vi "addcase.vi"() -> ()   [LabVIEW 2021]
uses:
  addcaase1.ctl
  addcase2.ctl
panel:
  out "train coming to point (500m before the cross)":i32
  out "speed of train":string
  out "Traffic":string
  out "Traffic condition":string
  out "train":string
  out "Number of Car 2":dbl
  out "Stop of traffic":i32
  out "Wait Time for Train":i32
  out "Number of Car":dbl
  in  "stop":bool
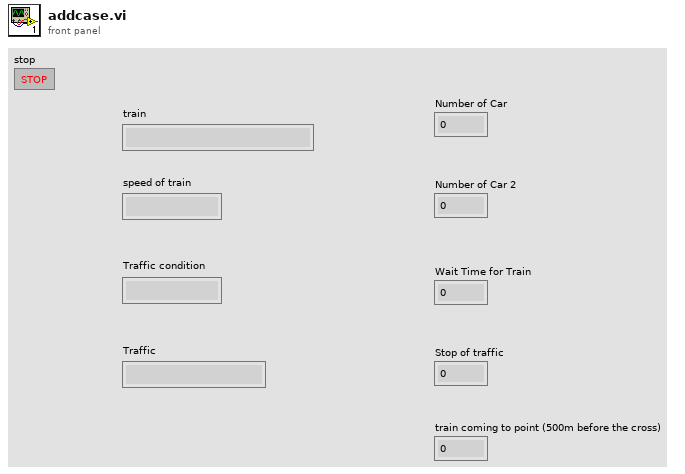
[diagram p1: front panel]
types:
  T1 = typedef "addcase2.ctl" = enum16{"Heavytraincrossing", "Heavytrafficwait", "Heavytraindepature", "Heavytrainwait", "Normal"}
  T2 = typedef "addcaase1.ctl" = enum16{"down", "traffice wait", "train departure", "up"}
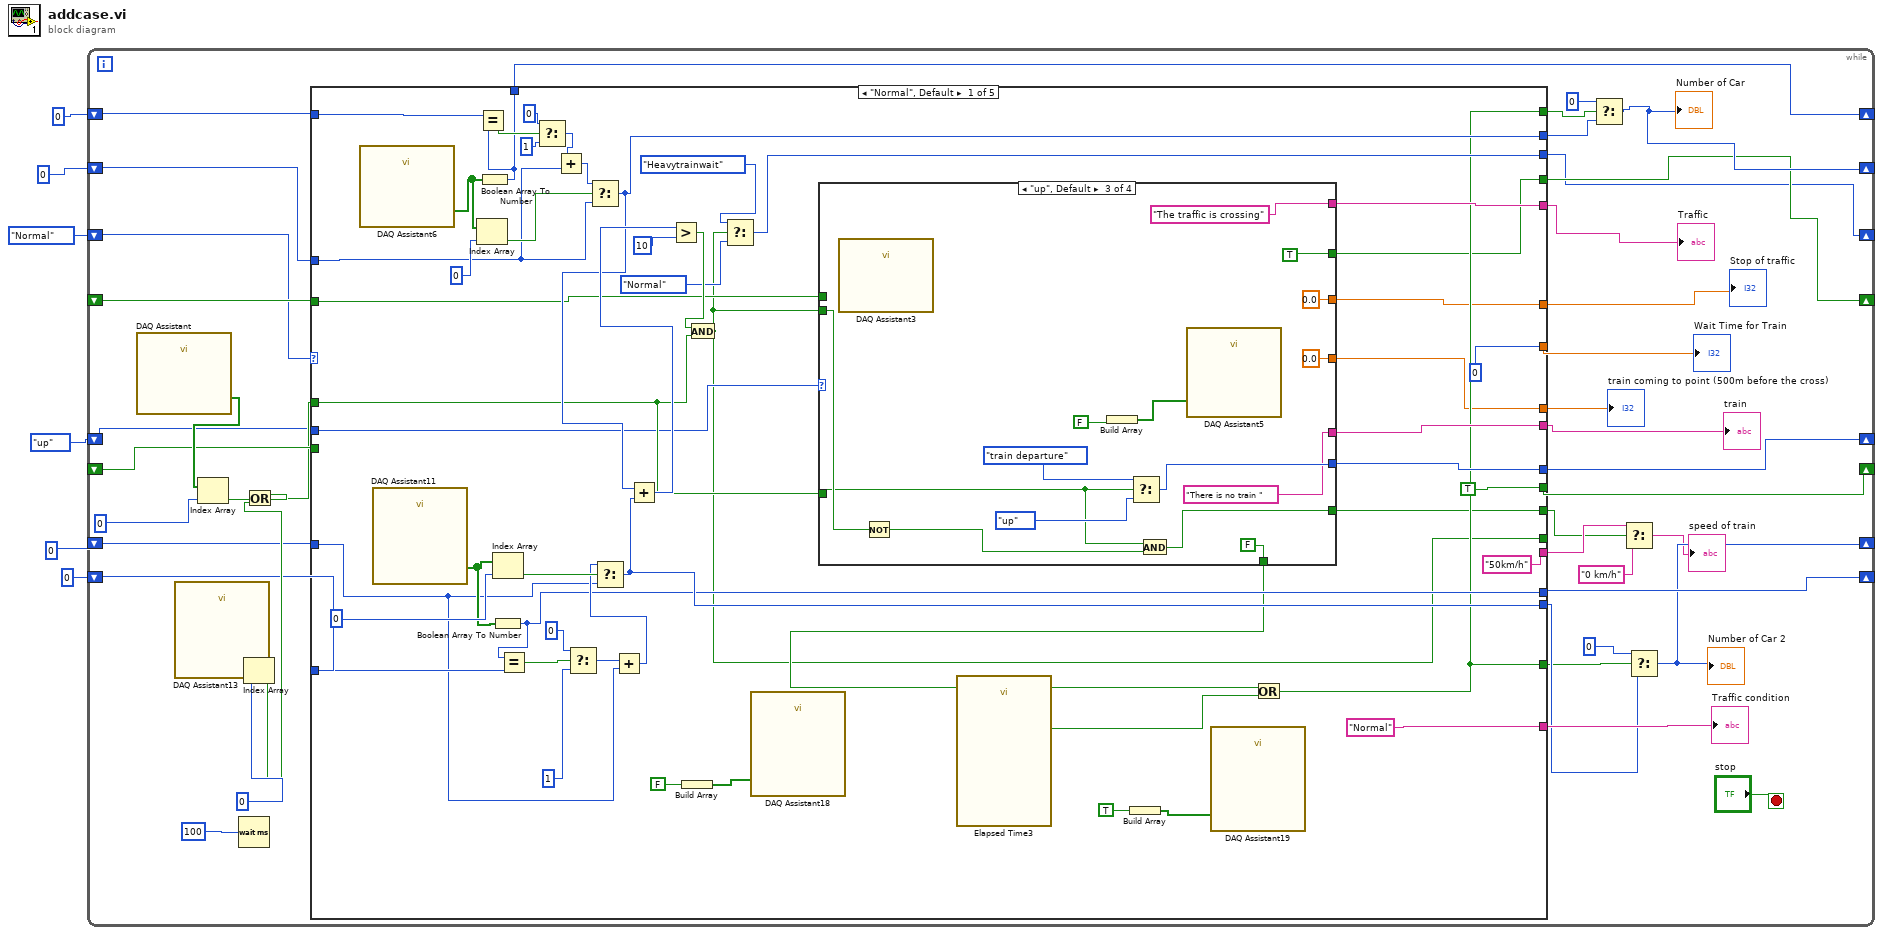
[diagram p0: block diagram]
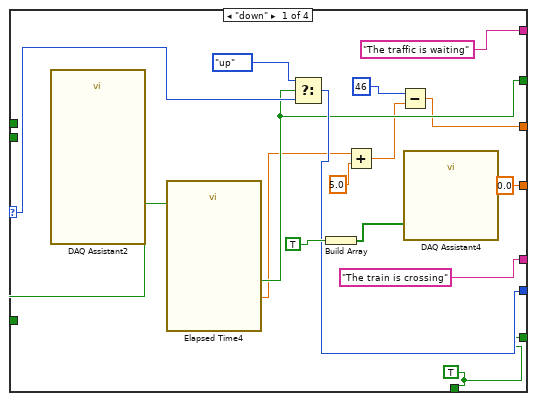
[diagram p2: hidden frame]
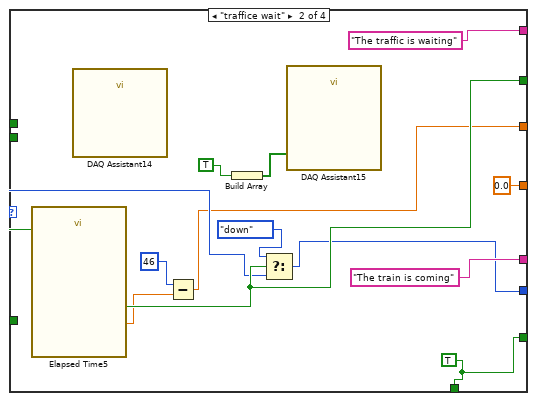
[diagram p3: hidden frame]
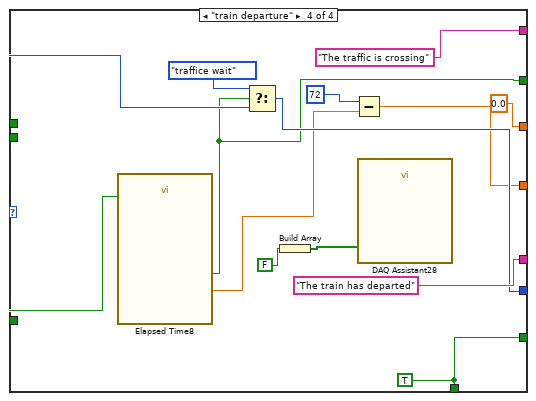
[diagram p4: hidden frame]
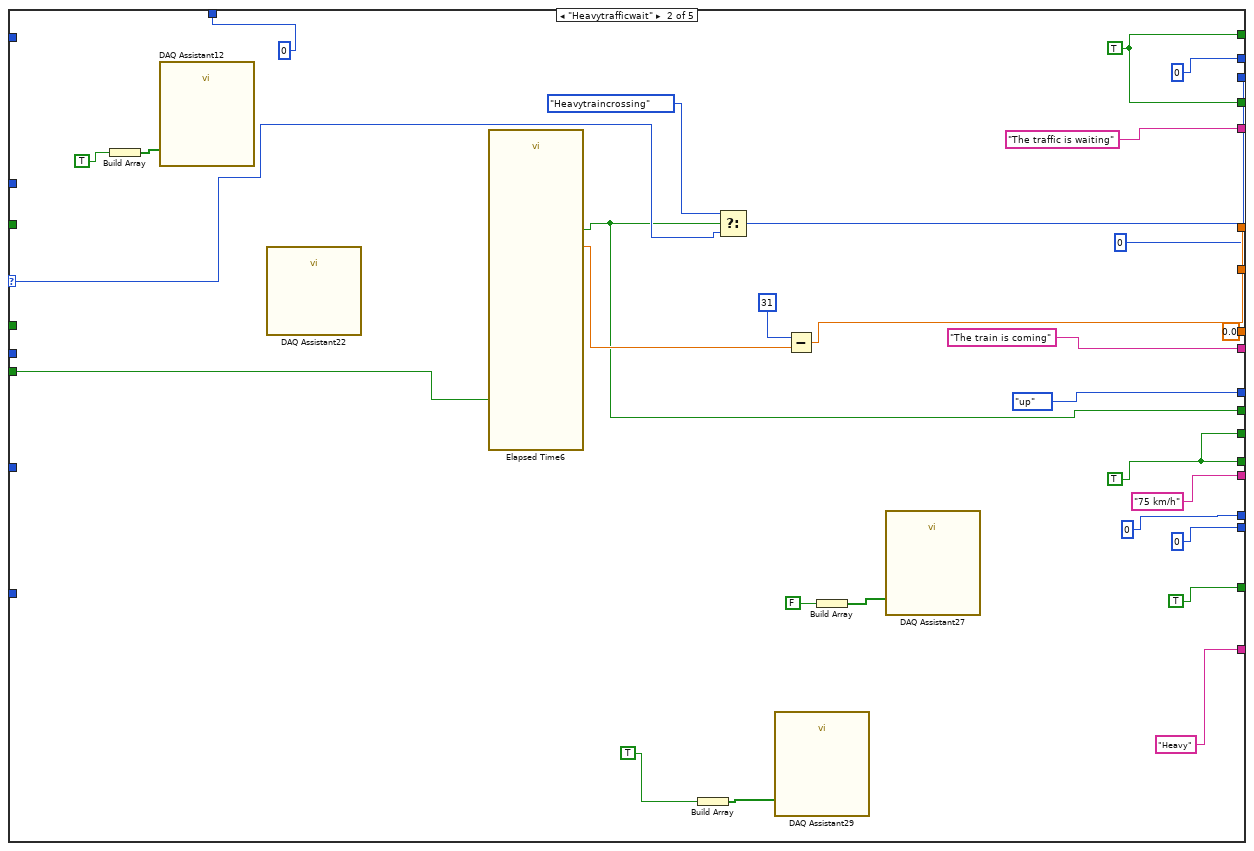
[diagram p5: hidden frame]
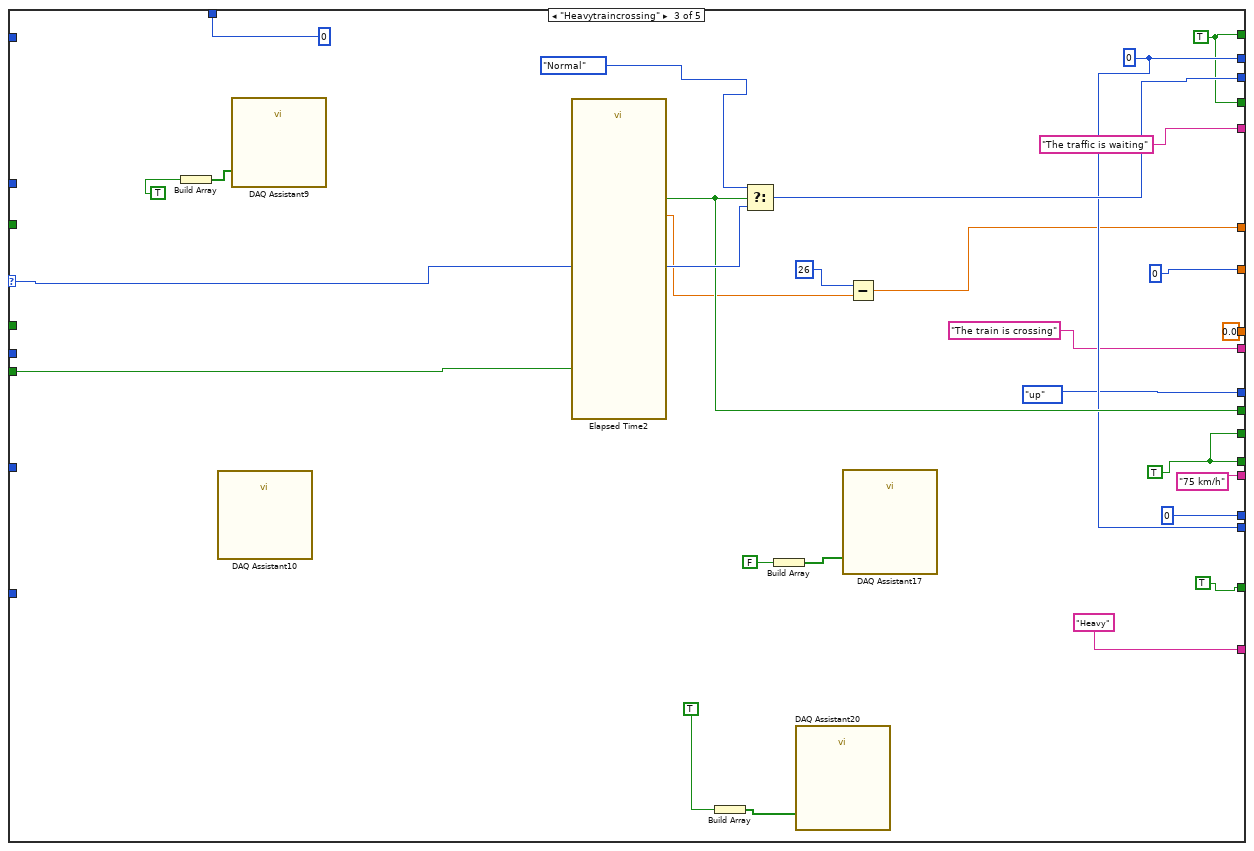
[diagram p6: hidden frame]
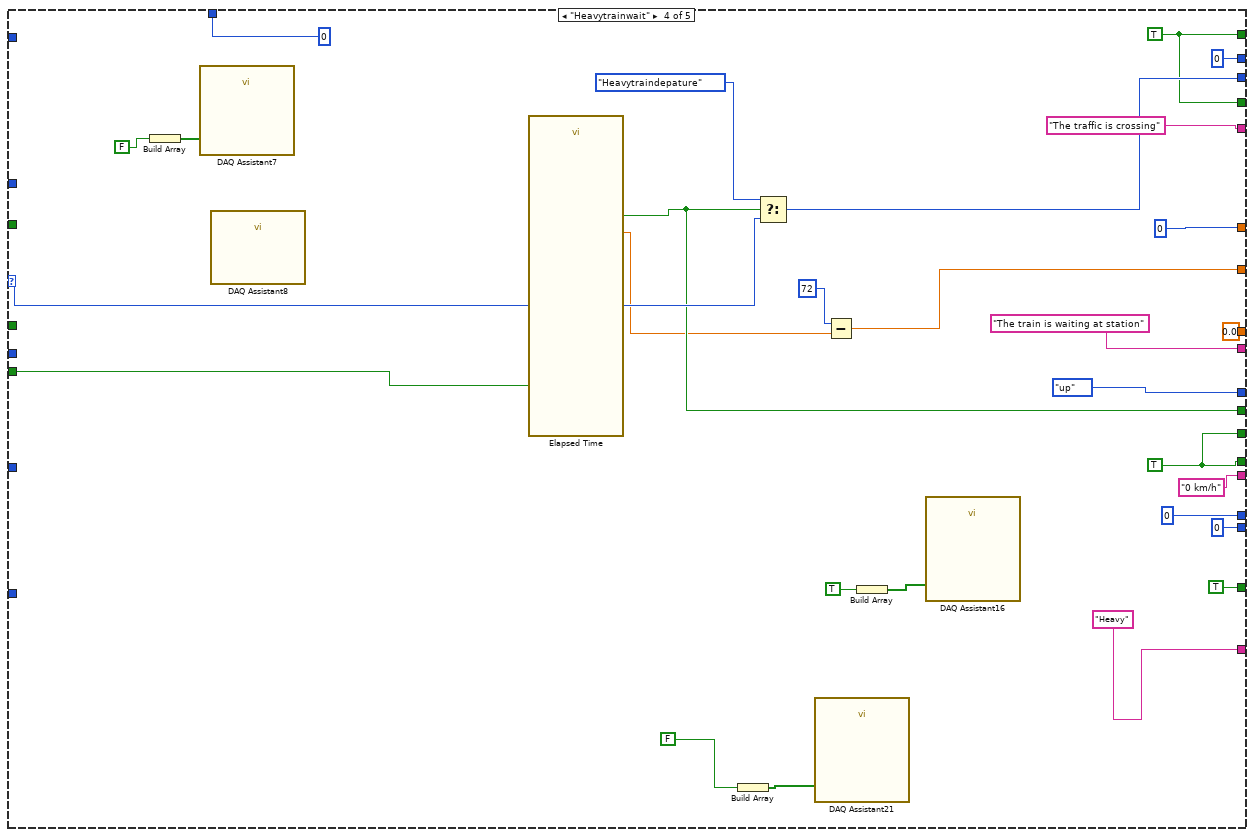
[diagram p7: hidden frame]
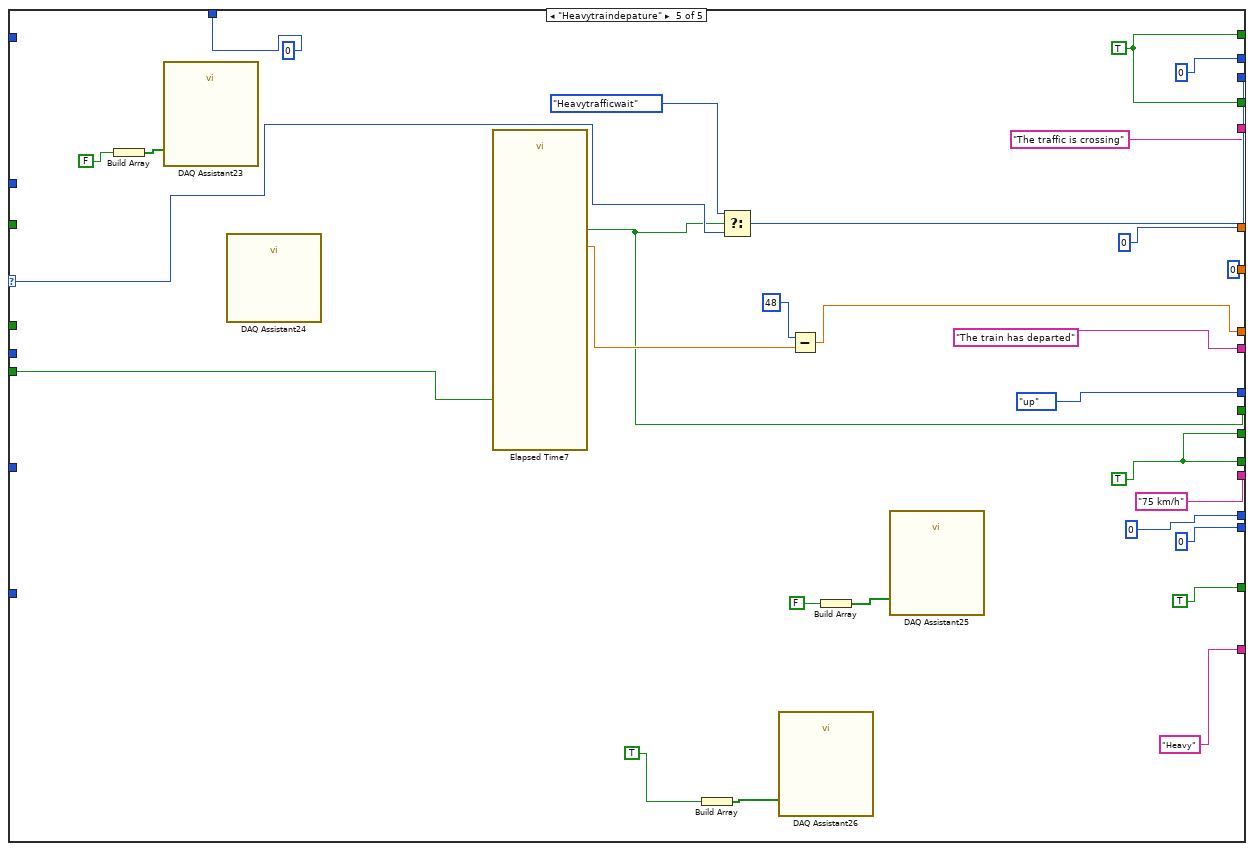
[diagram p8: hidden frame]
diagram:
  n1 = while {
    shift-right: [w22] -> _
    shift-left: 0 -> [w35]
    shift-right: [w42] -> _
    shift-left: _ -> [w41]
    shift-right: [w26] -> _
    shift-left: 0 -> [w34]
    shift-right: [w24] -> _
    shift-left: 0 ("index") -> [w33]
    shift-right: [w31] -> _
    shift-left: 0 ("index") -> [w32]
    shift-right: [w20] -> _
    shift-left: _ -> [w19]
    shift-right: [w14] -> _
    shift-left: addcaase1."up" -> [w15]
    shift-right: [w11] -> _
    shift-left: addcase2."Normal" -> [w12]
    stop <- "stop" stop-if-true
    n2 = call "DAQ Assistant"() -> ("data"=w46:bool[])  [unwired: 17 in, 2 out]
    n3 = call "DAQ Assistant13"() -> ("data"=w39:bool[])  [unwired: 17 in, 2 out]
    n4 = Index Array(array=w46, index=0) -> (element=w38:bool)
    n5 = Wait (ms)(milliseconds to wait=100) -> ()  [unwired: 1 out]
    n6 = Index Array(array=w39, index=0) -> (element=w37:bool)
    n7 = Or(x=w38, y=w37) -> (x .or. y?=w29:bool)
    n8 = case shown="\"Normal\", Default" w12 {
      selector: w12 -> [_ w175 w211 w239 w256]
      tunnel: w29 -> [w65 _ _ _ _]
      tunnel: [w98 w160 w210 w240 w255] -> w11
      tunnel: w35 -> [w78 _ _ _ _]
      tunnel: [w92 0 w206 0 0] -> w23
      tunnel: [w61 w167 w193 0 0] -> w44
      tunnel: [0 0 0 w221 0] -> w43
      tunnel: [TRUE w174 w208 w237 w254] -> w42
      tunnel: w41 -> [_ w177 w207 w236 w249]
      tunnel: w34 -> [w70 _ _ _ _]
      tunnel: [w93 0 w206 0 0] -> w27
      tunnel: w33 -> [w90 _ _ _ _]
      tunnel: [w85 u32 0 ("index") u32 0 ("index") u32 0 ("index") u32 0 ("index")] -> w24
      tunnel: [w84 addcaase1."up" addcaase1."up" addcaase1."up" addcaase1."up"] -> w14
      tunnel: w32 -> [w71 _ _ _ _]
      tunnel: [w72 u32 0 u32 0 u32 0 u32 0] -> w31
      tunnel: ["Normal" "Heavy" "Heavy" "Heavy" "Heavy"] -> w30
      tunnel: [w68 "The train is coming" "The train is crossing" "The train is waiting at station" "The train has departed"] -> w17
      tunnel: [w67 "The traffic is waiting" "The traffic is waiting" "The traffic is crossing" "The traffic is crossing"] -> w18
      tunnel: [w48 w159 w187 w214 w242] -> _
      tunnel: [w62 TRUE TRUE TRUE TRUE] -> w16
      tunnel: [w62 w163 w197 w225 w247] -> w21
      tunnel: [w60 w163 w197 w225 w247] -> w20
      tunnel: w19 -> [w59 _ _ _ _]
      tunnel: ["50km/h" "75 km/h" "75 km/h" "0 km/h" "75 km/h"] -> w10
      tunnel: w15 -> [w53 _ _ _ _]
      tunnel: [w52 0.0 ("Elapsed Time (s)") 0.0 ("Elapsed Time (s)") 0.0 ("Elapsed Time (s)") w244] -> w13
      tunnel: [w49 w159 w187 w214 w242] -> w8
      frame "Normal", Default {
        n9 = call "DAQ Assistant6"() -> ("data"=w88:bool[])  [unwired: 17 in, 2 out]
        n10 = call "DAQ Assistant11"() -> ("data"=w83:bool[])  [unwired: 17 in, 2 out]
        n11 = Index Array(array=w88, index=0) -> (element=w89:bool)
        n12 = Boolean Array To Number(Boolean array=w88) -> (number=w85:u32)
        n13 = Equal?(x=w90, y=w85) -> (x = y?=w87:bool)
        n14 = Index Array(array=w83, index=0) -> (element=w74:bool)
        n15 = Boolean Array To Number(Boolean array=w83) -> (number=w72:u32)
        n16 = Equal?(x=w72, y=w71) -> (x = y?=w82:bool)
        n17 = Select(t=0, s=w87, f=1) -> (s? t:f=w79:i32)
        n18 = Add(x=w79, y=w78) -> (x+y=w77:i32)
        n19 = Select(t=0, s=w82, f=1) -> (s? t:f=w75:i32)
        n20 = Select(t=w77, s=w89, f=w78) -> (s? t:f=w92:i32)
        n21 = Add(x=w75, y=w70) -> (x+y=w73:i32)
        n22 = Select(t=w73, s=w74, f=w70) -> (s? t:f=w93:i32)
        n23 = Add(x=w92, y=w93) -> (x+y=w94:i32)
        n24 = Greater?(x=w94, y=10) -> (0:w66:bool)
        n25 = Build Array(FALSE) -> (w58:bool[])
        n26 = And(x=w66, y=w65) -> (x .and. y?=w48:bool)
        n27 = Select(t=addcase2."Heavytrainwait", s=w48, f=addcase2."Normal") -> (s? t:f=w98:T1)
        n28 = call "DAQ Assistant18"("data"=w58) -> ()  [unwired: 17 in, 2 out]
        n29 = case shown="\"up\", Default" w53 {
          selector: w53 -> [w110 w123 _ w154]
          tunnel: w65 -> [_ _ w131 _]
          tunnel: [w109 w124 w143 w150] -> w84
          tunnel: ["The train is crossing" "The train is coming" "There is no train " "The train has departed"] -> w68
          tunnel: ["The traffic is waiting" "The traffic is waiting" "The traffic is crossing" "The traffic is crossing"] -> w67
          tunnel: [w100 w116 FALSE w145] -> w63
          tunnel: [w103 w119 0.0 ("Elapsed Time (s)") 0.0 ("Elapsed Time (s)")] -> w61
          tunnel: [w108 w125 TRUE w149] -> w60
          tunnel: w59 -> [w111 w126 _ w153]
          tunnel: [0.0 ("Elapsed Time (s)") 0.0 ("Elapsed Time (s)") 0.0 ("Elapsed Time (s)") w147] -> w52
          tunnel: [w100 w116 w130 w145] -> w49
          tunnel: w48 -> [_ _ w133 _]
          frame "down" {
            w100 = TRUE
            n30 = call "DAQ Assistant2"() -> ()  [unwired: 18 in, 2 out]
            n31 = call "Elapsed Time4"("Reset"=w111) -> ("Elapsed Time (s)"=w106:dbl, "Time has Elapsed"=w108:bool)  [unwired: 11 in, 6 out]
            n32 = Select(t=addcaase1."up", s=w108, f=w110) -> (s? t:f=w109:T2)
            n33 = Build Array(TRUE) -> (w115:bool[])
            n34 = Add(x=w106, y=5.0) -> (x+y=w104:dbl)
            n35 = Subtract(x=46, y=w104) -> (x-y=w103:dbl)
            n36 = call "DAQ Assistant4"("data"=w115) -> ()  [unwired: 17 in, 2 out]
          }
          frame "traffice wait" {
            w116 = TRUE
            n37 = call "Elapsed Time5"("Reset"=w126) -> ("Elapsed Time (s)"=w120:dbl, "Time has Elapsed"=w125:bool)  [unwired: 11 in, 6 out]
            n38 = call "DAQ Assistant14"() -> ()  [unwired: 18 in, 2 out]
            n39 = Subtract(x=46, y=w120) -> (x-y=w119:dbl)
            n40 = Build Array(TRUE) -> (w129:bool[])
            n41 = Select(t=addcaase1."down", s=w125, f=w123) -> (s? t:f=w124:T2)
            n42 = call "DAQ Assistant15"("data"=w129) -> ()  [unwired: 17 in, 2 out]
          }
          frame "up", Default {
            n43 = call "DAQ Assistant3"() -> ()  [unwired: 18 in, 2 out]
            n44 = Not(x=w133) -> (.not. x?=w132:bool)
            n45 = Build Array(FALSE) -> (w144:bool[])
            n46 = Select(t=addcaase1."train departure", s=w131, f=addcaase1."up") -> (s? t:f=w143:T2)
            n47 = And(x=w131, y=w132) -> (x .and. y?=w130:bool)
            n48 = call "DAQ Assistant5"("data"=w144) -> ()  [unwired: 17 in, 2 out]
          }
          frame "train departure" {
            w145 = TRUE
            n49 = call "Elapsed Time8"("Reset"=w153) -> ("Elapsed Time (s)"=w146:dbl, "Time has Elapsed"=w149:bool)  [unwired: 11 in, 6 out]
            n50 = Select(t=addcaase1."traffice wait", s=w149, f=w154) -> (s? t:f=w150:T2)
            n51 = Build Array(FALSE) -> (w158:bool[])
            n52 = Subtract(x=72, y=w146) -> (x-y=w147:dbl)
            n53 = call "DAQ Assistant28"("data"=w158) -> ()  [unwired: 17 in, 2 out]
          }
        }
        n54 = call "Elapsed Time3"() -> ("Time has Elapsed"=w64:bool)  [unwired: 12 in, 7 out]
        n55 = Build Array(TRUE) -> (w54:bool[])
        n56 = call "DAQ Assistant19"("data"=w54) -> ()  [unwired: 17 in, 2 out]
        n57 = Or(x=w63, y=w64) -> (x .or. y?=w62:bool)
      }
      frame "Heavytrafficwait" {
        w163 = TRUE
        w159 = TRUE
        n58 = Build Array(TRUE) -> (w186:bool[])
        n59 = call "DAQ Assistant12"("data"=w186) -> ()  [unwired: 17 in, 2 out]
        n60 = call "DAQ Assistant22"() -> ()  [unwired: 18 in, 2 out]
        n61 = call "Elapsed Time6"("Reset"=w177) -> ("Elapsed Time (s)"=w183:dbl, "Time has Elapsed"=w174:bool)  [unwired: 11 in, 6 out]
        n62 = Build Array(TRUE) -> (w184:bool[])
        n63 = Select(t=addcase2."Heavytraincrossing", s=w174, f=w175) -> (s? t:f=w160:T1)
        n64 = call "DAQ Assistant29"("data"=w184) -> ()  [unwired: 17 in, 2 out]
        n65 = Subtract(x=31, y=w183) -> (x-y=w167:dbl)
        n66 = Build Array(FALSE) -> (w185:bool[])
        n67 = call "DAQ Assistant27"("data"=w185) -> ()  [unwired: 17 in, 2 out]
      }
      frame "Heavytraincrossing" {
        w197 = TRUE
        w187 = TRUE
        w206 = 0
        n68 = Build Array(TRUE) -> (w212:bool[])
        n69 = call "DAQ Assistant10"() -> ()  [unwired: 18 in, 2 out]
        n70 = call "DAQ Assistant9"("data"=w212) -> ()  [unwired: 17 in, 2 out]
        n71 = call "Elapsed Time2"("Reset"=w207) -> ("Elapsed Time (s)"=w191:dbl, "Time has Elapsed"=w208:bool)  [unwired: 11 in, 6 out]
        n72 = Build Array(TRUE) -> (w195:bool[])
        n73 = Select(t=addcase2."Normal", s=w208, f=w211) -> (s? t:f=w210:T1)
        n74 = Build Array(FALSE) -> (w201:bool[])
        n75 = call "DAQ Assistant20"("data"=w195) -> ()  [unwired: 17 in, 2 out]
        n76 = call "DAQ Assistant17"("data"=w201) -> ()  [unwired: 17 in, 2 out]
        n77 = Subtract(x=26, y=w191) -> (x-y=w193:dbl)
      }
      frame "Heavytrainwait" {
        w225 = TRUE
        w214 = TRUE
        n78 = Build Array(FALSE) -> (w241:bool[])
        n79 = call "DAQ Assistant7"("data"=w241) -> ()  [unwired: 17 in, 2 out]
        n80 = call "DAQ Assistant8"() -> ()  [unwired: 18 in, 2 out]
        n81 = call "Elapsed Time"("Reset"=w236) -> ("Elapsed Time (s)"=w219:dbl, "Time has Elapsed"=w237:bool)  [unwired: 11 in, 6 out]
        n82 = Build Array(FALSE) -> (w222:bool[])
        n83 = Select(t=addcase2."Heavytraindepature", s=w237, f=w239) -> (s? t:f=w240:T1)
        n84 = call "DAQ Assistant21"("data"=w222) -> ()  [unwired: 17 in, 2 out]
        n85 = Subtract(x=72, y=w219) -> (x-y=w221:dbl)
        n86 = Build Array(TRUE) -> (w230:bool[])
        n87 = call "DAQ Assistant16"("data"=w230) -> ()  [unwired: 17 in, 2 out]
      }
      frame "Heavytraindepature" {
        w247 = TRUE
        w242 = TRUE
        n88 = Build Array(FALSE) -> (w269:bool[])
        n89 = call "DAQ Assistant23"("data"=w269) -> ()  [unwired: 17 in, 2 out]
        n90 = call "DAQ Assistant24"() -> ()  [unwired: 18 in, 2 out]
        n91 = call "Elapsed Time7"("Reset"=w249) -> ("Elapsed Time (s)"=w266:dbl, "Time has Elapsed"=w254:bool)  [unwired: 11 in, 6 out]
        n92 = Build Array(TRUE) -> (w267:bool[])
        n93 = Select(t=addcase2."Heavytrafficwait", s=w254, f=w256) -> (s? t:f=w255:T1)
        n94 = call "DAQ Assistant26"("data"=w267) -> ()  [unwired: 17 in, 2 out]
        n95 = Subtract(x=48, y=w266) -> (x-y=w244:dbl)
        n96 = Build Array(FALSE) -> (w268:bool[])
        n97 = call "DAQ Assistant25"("data"=w268) -> ()  [unwired: 17 in, 2 out]
      }
    }
    "Wait Time for Train" <- w43
    "Stop of traffic" <- w44
    "Traffic condition" <- w30
    "train" <- w17
    "Traffic" <- w18
    "train coming to point (500m before the cross)" <- w13
    n98 = Select(t=0, s=w21, f=w23) -> (s? t:f=w22:i32)
    "Number of Car" <- w22
    n99 = Select(t=w10, s=w8, f="0 km/h") -> (s? t:f=→"speed of train":string)
    n100 = Select(t=0, s=w16, f=w27) -> (s? t:f=w26:i32)
    "Number of Car 2" <- w26
  }
